vi "ECG AF sim.vi"() -> ()   [LabVIEW 2017]
uses:
  <vilib>/Platform/TimedLoop/XDataNode/wakeup.ctl
  <vilib>/Platform/TimedLoop/XDataNode/XDNodeRunTimeDep.lvlib
  <vilib>/Platform/TimedLoop/XDataNode/nitl_modes.ctl
  <vilib>/Platform/TimedLoop/XDataNode/timing_clust.ctl
  <vilib>/Platform/TimedLoop/XDataNode/XDataNode.xnode
  <vilib>/rvi/DataTransferAndStorage/Container/XNode/niFpgaContainer.xnode
  <vilib>/rvi/FIFO/Fifo_Resource/niFpgaFifoEmulationRefIn.vi
  <vilib>/rvi/LocalResourceManager/LocalResourceManager.xnode
  ECG Data.ctl
  Gradient Data.ctl
  IBP Data.ctl
  All Data.ctl
  <vilib>/eio/EIONode/EIONode.xnode
  <vilib>/rvi/DataTransferAndStorage/Container/Common/niFpgaContainerGetUniqueNameForEmu.vi
  <vilib>/rvi/DataTransferAndStorage/Container/Common/niFpgaContainerSetEmuInfo.vi
  <vilib>/rvi/eio/common/nirviEmuReportErrorAndStop.vi
  <vilib>/rvi/eio/common/nirviEmuTemplateMethod_errors.vi
  Trigger Params.ctl
  Channel Enum.ctl
panel:
  in  "Trigger":T1
  out "Send":bool
  in  "Reset":bool
  in  "stop":bool
  out "WeightSum":fxp<+/-,33,19> format="%.20g"
  out "BetaProduct":fxp<+/-,32,-1> format="%.33g"
  out "Number":u32
  in  "Filter Size":i16
  out "I In":i16
  out "II In":i16
  out "III In":i16
  out "aVR In":i16
  out "aVL In":i16
  out "aVF In":i16
  out "V1 In":i16
  out "V2 In":i16
  out "V3 In":i16
  out "V4 In":i16
  out "V5 In":i16
  out "V6 In":i16
  out "V4 Out":i16
  out "V5 Out":i16
  out "V6 Out":i16
  in  "Start 0":bool
  in  "Beta":fxp<+/-,32,-16>
  out "V3 Out":i16
  out "V2 Out":i16
  out "V1 Out":i16
  out "aVF Out":i16
  out "aVL Out":i16
  out "aVR Out":i16
  out "III Out":i16
  out "II Out":i16
  out "I Out":i16
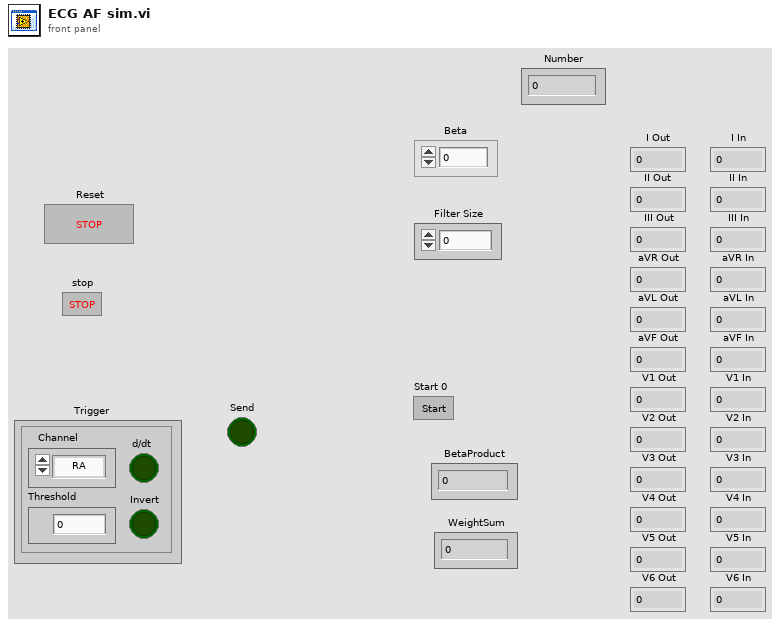
[diagram p1: front panel]
types:
  T1 = typedef "Trigger Params.ctl" = cluster{"Channel":T2, "Threshold":i16, "d/dt":bool, "Invert":bool}
  T2 = typedef "Channel Enum.ctl" = enum16{"RA", "LA", "LL", "V1", "V2", "V3", "V4", "V5", "V6", "I", "II", "III", "aVR", "aVL", "aVF", "Vw", "IBP1", "IBP2"}
  T3 = typedef "All Data.ctl" = cluster{"ECG":T4, "Gradients":T5, "IBP":T6}
  T4 = typedef "ECG Data.ctl" = cluster{"RA":fxp<+/-,16,16>, "LA":fxp<+/-,16,16>, "LL":fxp<+/-,16,16>, "V1":fxp<+/-,16,16>, "V2":fxp<+/-,16,16>, "V3":fxp<+/-,16,16>, "V4":fxp<+/-,16,16>, "V5":fxp<+/-,16,16>, "V6":fxp<+/-,16,16>}
  T5 = typedef "Gradient Data.ctl" = cluster{"X":fxp<+/-,16,16>, "Y":fxp<+/-,16,16>, "Z":fxp<+/-,16,16>}
  T6 = typedef "IBP Data.ctl" = cluster{"IBP0":fxp<+/-,16,16>, "IBP1":fxp<+/-,16,16>, "IBP2":fxp<+/-,16,16>}
  T7 = typedef "XDNodeRunTimeDep.lvlib/timing_clust.ctl" = cluster{"Expected End [f-1]":u64, "Actual End [f-1]":u64, "Finished Late? [f-1]":bool, "Expected End [i-1]":u64, "Actual End [i-1]":u64, "Finished Late? [i-1]":bool, "Expected Start [i]":u64, "Actual Start [i]":u64, "Expected Start [f]":u64, "Actual Start [f]":u64, "Source Name":string, "Structure Name":string, "Period":i64, "Deadline":i64, "Offset":i64, "Start":i64, "Priority":i32, "Timeout":i32, "Mode":T8, "Wakeup Reason":T9, "Error":errorcluster, "Source Type":string, "Secondary Source Type":string, "Global End Time":u64, "Global Start Time":u64, "Frame Duration":u64, "Iteration Duration":u64, "Assigned CPU":i32, "I/O Scan Engine Mode":u32}
  T8 = typedef "XDNodeRunTimeDep.lvlib/nitl_modes.ctl" = enum32{"No Change", "Process missed periods, maintain original phase", "Discard missed periods, maintain original phase", "Process missed periods, ignore original phase", "Discard missed periods, ignore original phase"}
  T9 = typedef "XDNodeRunTimeDep.lvlib/wakeup.ctl" = enum32{"Normal", "Aborted", "Asynchronous wakeup", "Timing source error", "Timed loop error", "Timeout"}
  T10 = typedef "Memory Block Channels.ctl" = cluster{"RA":T11, "LA":T11, "LL":T11, "V1":T11, "V2":T11, "V3":T11, "IBP0":T11, "IBP1":T11}
  T11 = typedef "MemoryBlocks.ctl" = cluster{"Taps":refnum<k21>, "Weights":refnum<k21>, "IO Weights":refnum<k21>, "IO Taps":refnum<k21>}
  T12 = cluster{"ECG":cluster{"RA":fxp<+/-,16,16>, "LA":fxp<+/-,16,16>, "LL":fxp<+/-,16,16>, "V1":fxp<+/-,16,16>, "V2":fxp<+/-,16,16>, "V3":fxp<+/-,16,16>, "V4":fxp<+/-,16,16>, "V5":fxp<+/-,16,16>, "V6":fxp<+/-,16,16>}, "Gradients":cluster{"X":fxp<+/-,16,16>, "Y":fxp<+/-,16,16>, "Z":fxp<+/-,16,16>}, "IBP":cluster{"IBP1":fxp<+/-,16,16>, "IBP2":fxp<+/-,16,16>, "IBP3":fxp<+/-,16,16>}}
  T13 = cluster{"BetaProduct":fxp<+/-,32,-1>, "WeightSum":fxp<+/-,33,19>}
  T14 = typedef "ECG Leads.ctl" = cluster{"RA":i16, "LA":i16, "LL":i16, "V1":i16, "V2":i16, "V3":i16, "V4":i16, "V5":i16, "Trigger":i16, "I":i16, "II":i16, "III":i16, "aVR":i16, "aVL":i16, "aVF":i16, "Vw":i16}
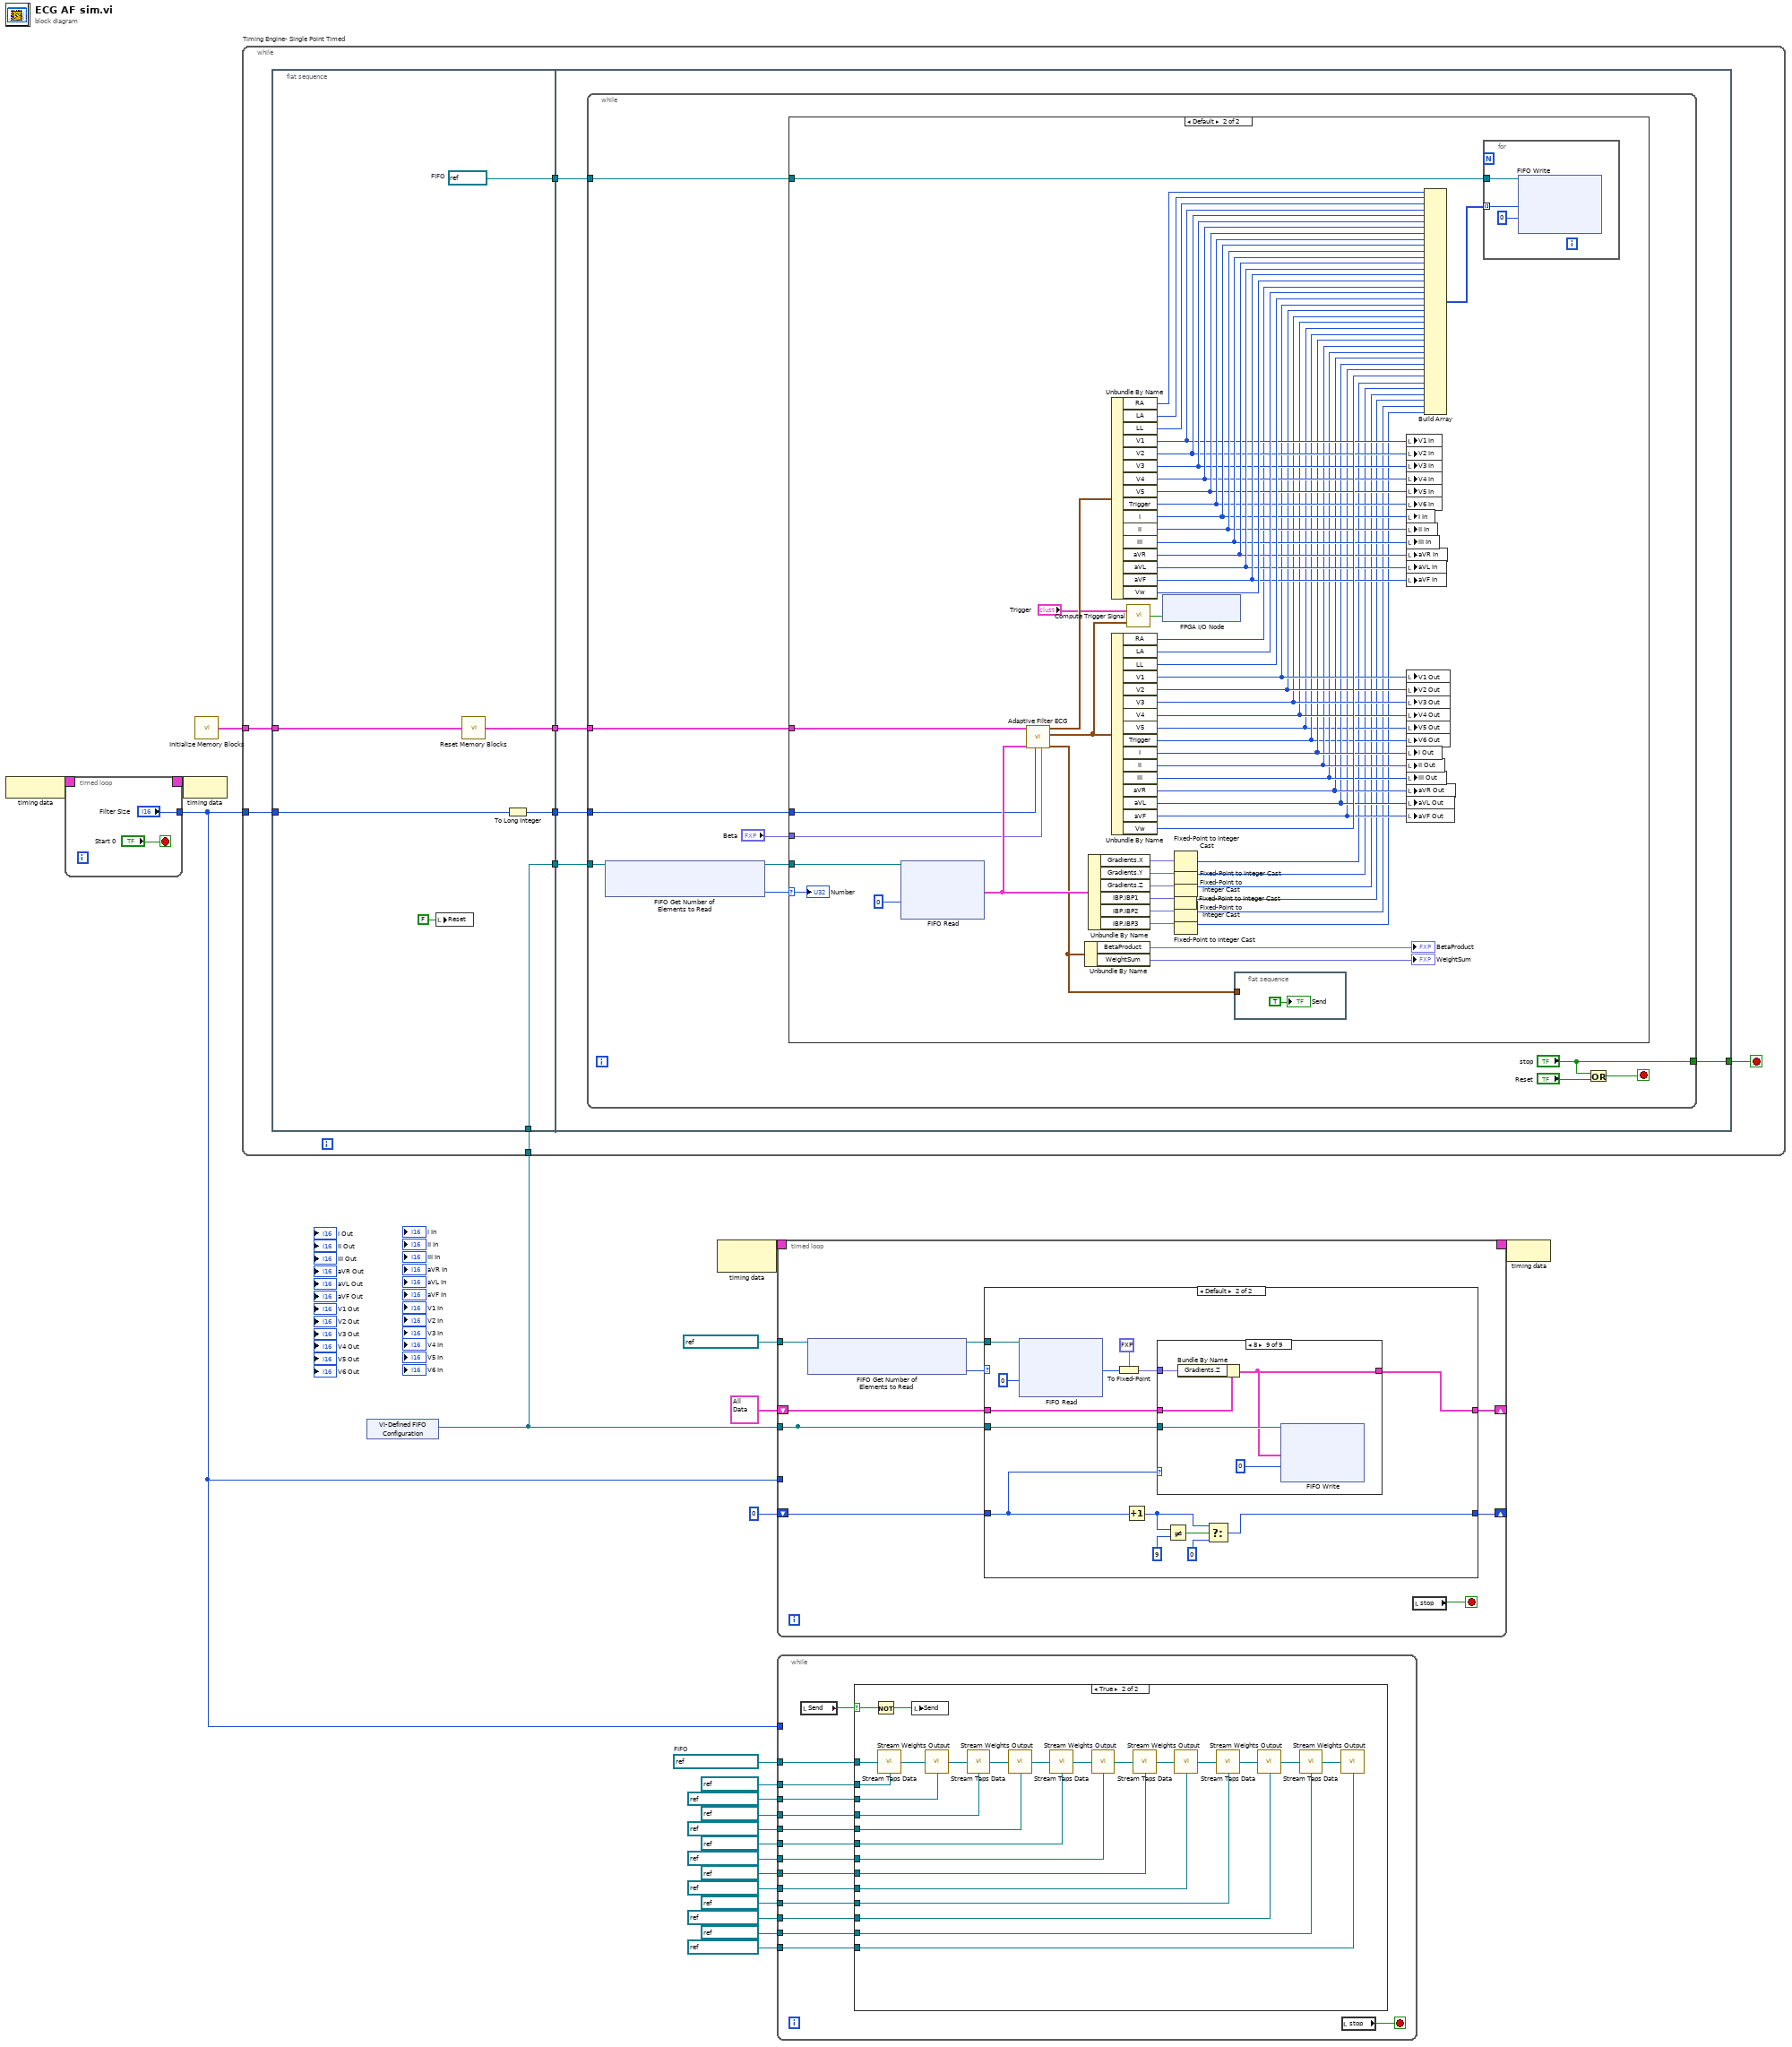
[diagram p0: block diagram]
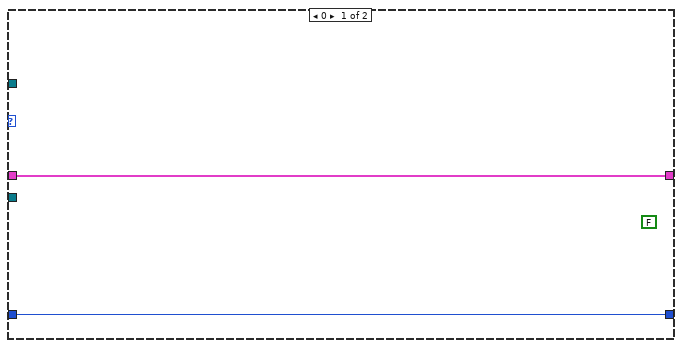
[diagram p3: hidden frame]
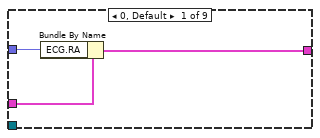
[diagram p4: hidden frame]
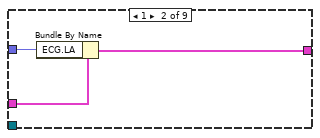
[diagram p5: hidden frame]
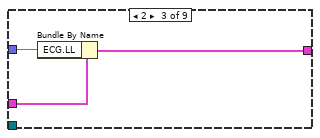
[diagram p6: hidden frame]
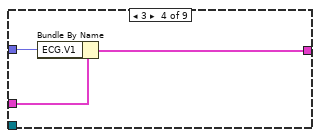
[diagram p7: hidden frame]
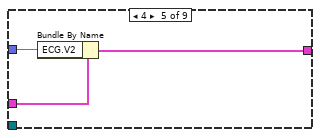
[diagram p8: hidden frame]
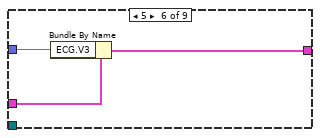
[diagram p9: hidden frame]
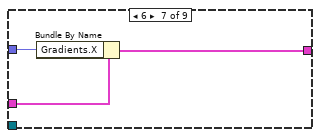
[diagram p10: hidden frame]
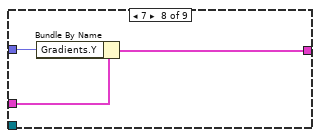
[diagram p11: hidden frame]
diagram:
  w18 = refnum<k21> "FIFO Filter Specs"  # FIFO
  n1 = node-c288 ("Input Node")() -> (w3:T7)
  n2 = timed-loop "initWait" {
    timing: w3 -> [_]
    timing-out: [_] -> w2
    tunnel: ["Filter Size"] -> w1
    stop <- "Start 0" stop-if-true
  }
  n3 = node-c288 ("Output Node")(w2) -> ()
  n4 = call "Initialize Memory Blocks.vi"() -> ("Memory"=w5:T10)
  n5 = xnode "VI-Defined FIFO Configuration"() -> ("FIFO Out"=w19:refnum<k21>)
  n6 = while "Timing Engine- Single Point Timed" {
    tunnel: w19 -> [w31]
    tunnel: w5 -> [w29]
    tunnel: w1 -> [w28]
    stop <- w30 stop-if-true
    n7 = flat-sequence "MainSeq" {
      tunnel: [w42] -> w35
      tunnel: [w40] -> w34
      tunnel: [w39] -> w33
      tunnel: [w41] -> w32
      tunnel: w31 -> [w39]
      tunnel: w29 -> [w38]
      tunnel: w28 -> [w37]
      tunnel: w35 -> [w47]
      tunnel: w34 -> [w46]
      tunnel: w33 -> [w45]
      tunnel: w32 -> [w44]
      tunnel: [w43] -> w30
      frame #0 {
        w42 = refnum<k21> "FIFO"  # FIFO
        n8 = local write "Reset"(FALSE ("Reset")) -> ()
        n9 = call "Reset Memory Blocks.vi"("Memory Blocks In"=w38) -> ("Memory Blocks Out"=w41:T10)  [unwired: 1 in]
        n10 = To Long Integer(number=w37) -> (32bit integer=w40:i32)
      }
      frame #1 {
        n11 = while {
          tunnel: w45 -> [w57]
          tunnel: w47 -> [w54]
          tunnel: w46 -> [w52]
          tunnel: w44 -> [w48]
          tunnel: ["stop"] -> w43
          stop <- w51 stop-if-true
          n12 = xnode ("FIFO Get Number of Elements to Read")("FIFO In"=w57) -> ("Number of Elements to Read"=w53:u32, "FIFO Out"=w56:refnum<k21>)
          n13 = case shown="Default" w53 {
            selector: w53 -> [_ w83]
            tunnel: w56 -> [_ w117]
            tunnel: "Beta" -> [_ w72]
            tunnel: w54 -> [_ w115]
            tunnel: w52 -> [_ w73]
            tunnel: w48 -> [_ w75]
            frame 0 {
            }
            frame Default {
              n14 = xnode ("FIFO Read")("Timeout"=0, "FIFO In"=w117) -> ("Element"=w74:T12)  [unwired: 2 out]
              n15 = call "Adaptive Filter ECG.vi"("Beta"=w72, "Filter Length"=w73, "Data in"=w74, "Memory Blocks In"=w75) -> ("Data"=w71:T13, "Filtered Leads"=w59:T14, "Raw Leads"=w70:T14)  [unwired: 4 in, 1 out]
              n16 = Unbundle By Name(w71) -> ("BetaProduct"=→"BetaProduct":fxp<+/-,32,-1>, "WeightSum"=→"WeightSum":fxp<+/-,33,19>)
              n17 = Unbundle By Name(w74) -> ("Gradients.X"=w82:fxp<+/-,16,16>, "Gradients.Y"=w81:fxp<+/-,16,16>, "Gradients.Z"=w80:fxp<+/-,16,16>, "IBP.IBP1"=w66:fxp<+/-,16,16>, "IBP.IBP2"=w65:fxp<+/-,16,16>, "IBP.IBP3"=w64:fxp<+/-,16,16>)
              n18 = Unbundle By Name(w70) -> ("RA"=w79:i16, "LA"=w113:i16, "LL"=w112:i16, "V1"=w96:i16, "V2"=w97:i16, "V3"=w98:i16, "V4"=w99:i16, "V5"=w100:i16, "Trigger"=w101:i16, "I"=w102:i16, "II"=w103:i16, "III"=w104:i16, "aVR"=w105:i16, "aVL"=w106:i16, "aVF"=w107:i16, "Vw"=w111:i16)
              n19 = Unbundle By Name(w59) -> ("RA"=w78:i16, "LA"=w110:i16, "LL"=w109:i16, "V1"=w95:i16, "V2"=w94:i16, "V3"=w93:i16, "V4"=w92:i16, "V5"=w84:i16, "Trigger"=w85:i16, "I"=w91:i16, "II"=w90:i16, "III"=w89:i16, "aVR"=w88:i16, "aVL"=w87:i16, "aVF"=w86:i16, "Vw"=w108:i16)
              n20 = call "Compute Trigger Signal.vi"("Leads"=w59, "Trigger"="Trigger") -> ("Trigger Out"=w58:bool)
              n21 = xnode "FPGA I/O Node"("Trigger Out"=w58) -> ()  [unwired: 1 in, 1 out]
              n22 = Fixed-Point to Integer Cast(1:w66) -> (0:w63:i16)
              n23 = Fixed-Point to Integer Cast(1:w82) -> (0:w69:i16)
              n24 = Fixed-Point to Integer Cast(1:w81) -> (0:w68:i16)
              n25 = Fixed-Point to Integer Cast(1:w80) -> (0:w67:i16)
              n26 = Fixed-Point to Integer Cast(1:w65) -> (0:w62:i16)
              n27 = Fixed-Point to Integer Cast(1:w64) -> (0:w61:i16)
              n28 = flat-sequence {
                tunnel: w71 -> [_]
                frame #0 {
                  "Send" <- TRUE ("Send")
                }
              }
              n29 = local write "V1 In"(w96) -> ()
              n30 = local write "V2 In"(w97) -> ()
              n31 = local write "V3 In"(w98) -> ()
              n32 = local write "V4 In"(w99) -> ()
              n33 = local write "V5 In"(w100) -> ()
              n34 = local write "V6 In"(w101) -> ()
              n35 = local write "I In"(w102) -> ()
              n36 = local write "II In"(w103) -> ()
              n37 = local write "III In"(w104) -> ()
              n38 = local write "aVR In"(w105) -> ()
              n39 = local write "aVL In"(w106) -> ()
              n40 = local write "aVF In"(w107) -> ()
              n41 = local write "V1 Out"(w95) -> ()
              n42 = local write "V2 Out"(w94) -> ()
              n43 = local write "V3 Out"(w93) -> ()
              n44 = local write "V4 Out"(w92) -> ()
              n45 = local write "V5 Out"(w84) -> ()
              n46 = local write "V6 Out"(w85) -> ()
              n47 = local write "I Out"(w91) -> ()
              n48 = local write "II Out"(w90) -> ()
              n49 = local write "III Out"(w89) -> ()
              n50 = local write "aVR Out"(w88) -> ()
              n51 = local write "aVL Out"(w87) -> ()
              n52 = local write "aVF Out"(w86) -> ()
              n53 = Build Array(w79, w113, w112, w96, w97, w98, w99, w100, w101, w102, w103, w104, w105, w106, w107, w111, w78, w110, w109, w95, w94, w93, w92, w84, w85, w91, w90, w89, w88, w87, w86, w108, w69, w68, w67, w63, w62, w61) -> (w114:i16[])
              n54 = for {
                tunnel: w115 -> [w121]
                tunnel: w114 -> [w119] mode=indexing
                n55 = xnode ("FIFO Write")("Element"=w119, "Timeout"=0, "FIFO In"=w121) -> ()  [unwired: 2 out]
              }
              "Number" <- w83
            }
          }
          n56 = Or(x="stop", y="Reset") -> (x .or. y?=w51:bool)
        }
      }
    }
  }
  n57 = node-c288() -> (w23:T7)  [unwired: 1 in]
  n58 = timed-loop {
    timing: w23 -> [_]
    timing-out: [_] -> w22
    tunnel: refnum<k21> "FIFO Simulate" ("FIFO Out") -> [w131]
    shift-right: [w128] -> _
    shift-left: i16 0 -> [w129]
    shift-right: [w125] -> _
    shift-left: T3 {"ECG"={"RA"=0.0, "LA"=0.0, "LL"=0.0, "V1"=0.0, "V2"=0.0, "V3"=0.0, "V4"=0.0, "V5"=0.0, "V6"=0.0}, "Gradients"={"X"=0.0, "Y"=0.0, "Z"=0.0}, "IBP"={"IBP0"=0.0, "IBP1"=0.0, "IBP2"=0.0}} ("Data") -> [w126]
    tunnel: [w124] -> _
    tunnel: w19 -> [w124]
    tunnel: [w122] -> _
    tunnel: w1 -> [w122]
    stop <- w123 stop-if-true
    n59 = xnode ("FIFO Get Number of Elements to Read")("FIFO In"=w131) -> ("Number of Elements to Read"=w130:u32, "FIFO Out"=w127:refnum<k21>)
    n60 = case shown="Default" w130 {
      tunnel: w129 -> [w133 w140]
      tunnel: [w133 w143] -> w128
      tunnel: w127 -> [_ w142]
      tunnel: w126 -> [w132 w138]
      tunnel: [w132 w137] -> w125
      tunnel: w124 -> [_ w136]
      frame 0 {
        (unwired) FALSE
      }
      frame Default {
        n61 = xnode ("FIFO Read")("Timeout"=0, "FIFO In"=w142) -> ("Element"=w139:i16)  [unwired: 2 out]
        n62 = To Fixed-Point(fixed-point type=fxp<+/-,16,16> 0.0, number=w139) -> (fixed-point=w135:fxp<+/-,16,16>)
        n63 = Increment(x=w140) -> (x+1=w145:i16)
        n64 = case shown="8" w140 {
          tunnel: w135 -> [w149 w152 w155 w158 w161 w164 w167 w170 w175]
          tunnel: w138 -> [w150 w153 w156 w159 w162 w165 w168 w171 w176]
          tunnel: [w148 w151 w154 w157 w160 w163 w166 w169 w172] -> w137
          tunnel: w136 -> [_ _ _ _ _ _ _ _ w174]
          frame 0, Default {
            n65 = Bundle By Name(cluster=w150, "ECG.RA"=w149) -> (w148:T3)
          }
          frame 1 {
            n66 = Bundle By Name(cluster=w153, "ECG.LA"=w152) -> (w151:T3)
          }
          frame 2 {
            n67 = Bundle By Name(cluster=w156, "ECG.LL"=w155) -> (w154:T3)
          }
          frame 3 {
            n68 = Bundle By Name(cluster=w159, "ECG.V1"=w158) -> (w157:T3)
          }
          frame 4 {
            n69 = Bundle By Name(cluster=w162, "ECG.V2"=w161) -> (w160:T3)
          }
          frame 5 {
            n70 = Bundle By Name(cluster=w165, "ECG.V3"=w164) -> (w163:T3)
          }
          frame 6 {
            n71 = Bundle By Name(cluster=w168, "Gradients.X"=w167) -> (w166:T3)
          }
          frame 7 {
            n72 = Bundle By Name(cluster=w171, "Gradients.Y"=w170) -> (w169:T3)
          }
          frame 8 {
            n73 = Bundle By Name(cluster=w176, "Gradients.Z"=w175) -> (w172:T3)
            n74 = xnode ("FIFO Write")("Element"=w172, "Timeout"=0, "FIFO In"=w174) -> ()  [unwired: 2 out]
          }
        }
        n75 = Not Equal?(x=w145, y=i16 9) -> (x != y?=w146:bool)
        n76 = Select(t=w145, s=w146, f=i16 0) -> (s? t:f=w143:i16)
      }
    }
    n77 = local read "stop"() -> (w123:bool)
  }
  n78 = while {
    tunnel: w18 -> [w192]
    tunnel: refnum<k21> "IO Taps 0" ("Memory") -> [w191]
    tunnel: refnum<k21> "IO Weights 0" ("Memory In") -> [w190]
    tunnel: refnum<k21> "IO Taps 1" ("Memory") -> [w189]
    tunnel: refnum<k21> "IO Weights 1" ("Memory In") -> [w188]
    tunnel: refnum<k21> "IO Taps 2" ("Memory") -> [w187]
    tunnel: refnum<k21> "IO Weights 2" ("Memory In") -> [w186]
    tunnel: refnum<k21> "IO Taps 3" ("Memory") -> [w185]
    tunnel: refnum<k21> "IO Weights 3" ("Memory In") -> [w184]
    tunnel: refnum<k21> "IO Taps 4" ("Memory") -> [w183]
    tunnel: refnum<k21> "IO Weights 4" ("Memory In") -> [w182]
    tunnel: refnum<k21> "IO Taps 5" ("Memory") -> [w181]
    tunnel: refnum<k21> "IO Weights 5" ("Memory In") -> [w180]
    tunnel: w1 -> [_]
    stop <- w179 stop-if-true
    n79 = local read "Send"() -> (w193:bool)
    n80 = case shown="True" w193 {
      selector: w193 -> [_ w219]
      tunnel: w192 -> [_ w217]
      tunnel: w191 -> [_ w215]
      tunnel: w190 -> [_ w214]
      tunnel: w189 -> [_ w211]
      tunnel: w188 -> [_ w210]
      tunnel: w187 -> [_ w208]
      tunnel: w186 -> [_ w207]
      tunnel: w185 -> [_ w203]
      tunnel: w184 -> [_ w202]
      tunnel: w183 -> [_ w197]
      tunnel: w182 -> [_ w196]
      tunnel: w181 -> [_ w195]
      tunnel: w180 -> [_ w194]
      frame False {
      }
      frame True {
        n81 = Not(x=w219) -> (.not. x?=w218:bool)
        n82 = call "Stream Taps Data.vi"("FIFO In"=w217, "Memory"=w215) -> ("FIFO out"=w216:refnum<k21>)
        n83 = local write "Send"(w218) -> ()
        n84 = call "Stream Weights Output.vi"("FIFO in"=w216, "Memory In"=w214) -> ("FIFO out"=w212:refnum<k21>)
        n85 = call "Stream Taps Data.vi"("FIFO In"=w212, "Memory"=w211) -> ("FIFO out"=w213:refnum<k21>)
        n86 = call "Stream Weights Output.vi"("FIFO in"=w213, "Memory In"=w210) -> ("FIFO out"=w209:refnum<k21>)
        n87 = call "Stream Taps Data.vi"("FIFO In"=w209, "Memory"=w208) -> ("FIFO out"=w206:refnum<k21>)
        n88 = call "Stream Weights Output.vi"("FIFO in"=w206, "Memory In"=w207) -> ("FIFO out"=w205:refnum<k21>)
        n89 = call "Stream Taps Data.vi"("FIFO In"=w205, "Memory"=w203) -> ("FIFO out"=w204:refnum<k21>)
        n90 = call "Stream Weights Output.vi"("FIFO in"=w204, "Memory In"=w202) -> ("FIFO out"=w198:refnum<k21>)
        n91 = call "Stream Taps Data.vi"("FIFO In"=w198, "Memory"=w197) -> ("FIFO out"=w199:refnum<k21>)
        n92 = call "Stream Weights Output.vi"("FIFO in"=w199, "Memory In"=w196) -> ("FIFO out"=w200:refnum<k21>)
        n93 = call "Stream Taps Data.vi"("FIFO In"=w200, "Memory"=w195) -> ("FIFO out"=w201:refnum<k21>)
        n94 = call "Stream Weights Output.vi"("FIFO in"=w201, "Memory In"=w194) -> ()  [unwired: 1 out]
      }
    }
    n95 = local read "stop"() -> (w179:bool)
  }
  n96 = node-c288(w22) -> ()
